vi "保存CSV数据.vi"(8 "路径":path, 11 "数据":sgl[][](array[numeric])) -> ()   [LabVIEW 2016]
uses:
  <vilib>/Utility/file.llb/Write To Spreadsheet File (DBL).vi
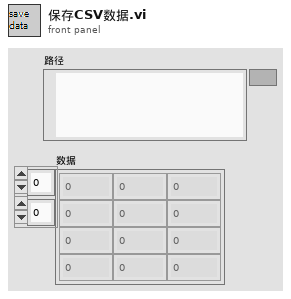
[diagram p1: front panel]
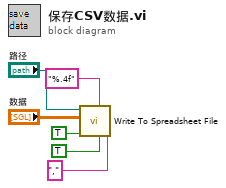
[diagram p0: block diagram]
diagram:
  n1 = call-poly <vilib>:"Write To Spreadsheet File.vi"("delimiter (\\t)"="," ("delimiter (\\t)"), "transpose? (no:F)"=TRUE, "format (%.3f)"="%.4f", "append to file? (new file:F)"=TRUE, "2D data"="数据", "file path (dialog if empty)"="路径") -> ()  [unwired: 2 in, 1 out]
